vi "SetandReadIVIsamplePowersupply.vi"(3 "error in (no error)":errorcluster, 4 "level (0.0 Volts)":dbl format="%.2f", 5 "channel name (\"CHANNEL1\")":string="CHANNEL1", 6 "instrument handle":refnum<k15>) -> (0 "error out":errorcluster, 1 "measurement":dbl format="%.2f", 2 "instrument handle out":refnum<k15>)   [LabVIEW 2013]
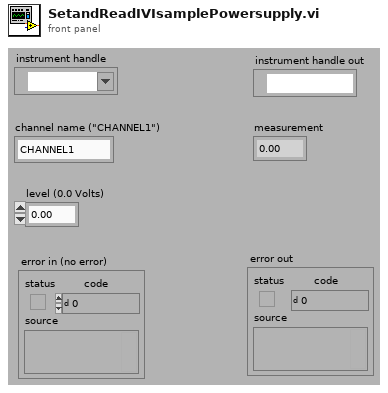
[diagram p1: front panel]
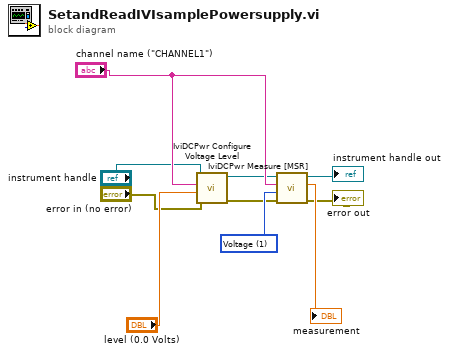
[diagram p0: block diagram]
diagram:
  w10 = 1 items=["Voltage"=1, "Current"=0] ("measurement type (voltage)")
  n1 = call <vilib>:"IviDCPwr Configure Voltage Level.vi"("error in (no error)"="error in (no error)", "level (0.0 Volts)"="level (0.0 Volts)", "channel name (\"CHANNEL1\")"="channel name (\"CHANNEL1\")", "instrument handle"="instrument handle") -> ("error out"=w9:errorcluster, "instrument handle out"=w1:refnum<k15>)  [unwired: 6 out]
  n2 = call <vilib>:"IviDCPwr Measure [MSR].vi"("error in (no error)"=w9, "measurement type (voltage)"=w10, "channel name (\"CHANNEL1\")"="channel name (\"CHANNEL1\")", "instrument handle"=w1) -> ("error out"=→"error out":errorcluster, "measurement"=→"measurement":dbl, "instrument handle out"=→"instrument handle out":refnum<k15>)  [unwired: 5 out]
